vi "Get State.vi"(8 "error in (no error)":errorcluster, 11 "Spectrum Recorder in":refnum<class "Spectrum Recorder.lvclass">) -> (0 "error out":errorcluster, 3 "Spectrum Recorder out":refnum<class "Spectrum Recorder.lvclass">)   [LabVIEW 2016, in "Spectrum Recorder.lvclass"]
uses:
  Spectrum Recorder.lvclass
  Spectrum Recorder.lvclass/Spectrum Recorder.ctl
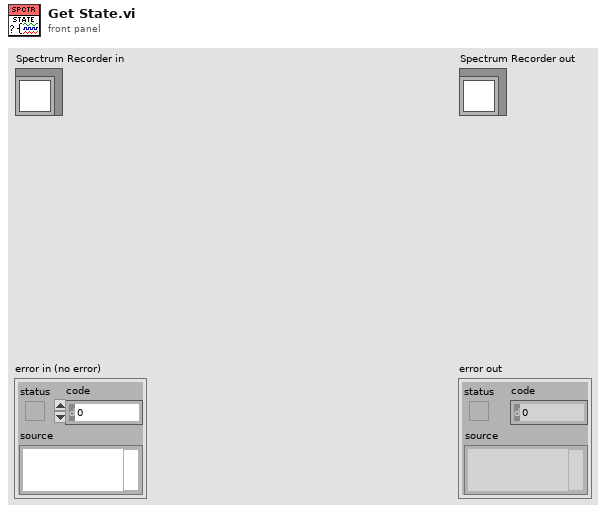
[diagram p1: front panel]
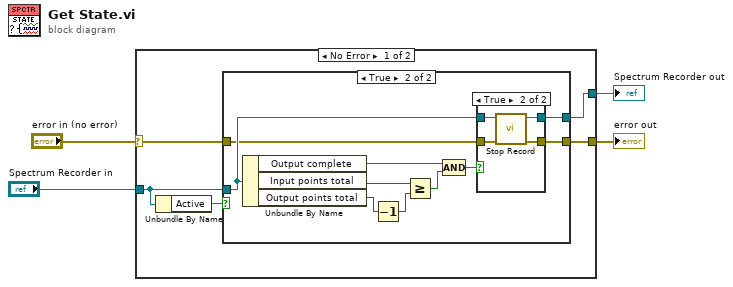
[diagram p0: block diagram]
diagram:
  n1 = case shown="No Error" "error in (no error)" {
    selector: "error in (no error)" -> [w6 w29]
    tunnel: [w5 w29] -> w3
    tunnel: [w7 w28] -> w1
    tunnel: "Spectrum Recorder in" -> [w8 w28]
    frame No Error {
      n2 = Unbundle By Name(w8) -> ("Active"=w9:bool)
      n3 = case shown="True" w9 {
        tunnel: w8 -> [w10 w17]
        tunnel: w6 -> [w11 w16]
        tunnel: [w11 w15] -> w5
        tunnel: [w10 w14] -> w7
        frame False {
        }
        frame True {
          n4 = Unbundle By Name(w17) -> ("Output complete"=w12:bool, "Input points total"=w20:i64, "Output points total"=w19:i64)
          n5 = Decrement(x=w19) -> (x-1=w13:i64)
          n6 = Greater Or Equal?(x=w20, y=w13) -> (x >= y?=w18:bool)
          n7 = Compound Arithmetic op=AND(w12, w18) -> (w21:bool)
          n8 = case shown="True" w21 {
            tunnel: w17 -> [w23 w27]
            tunnel: w16 -> [w22 w26]
            tunnel: [w22 w25] -> w15
            tunnel: [w23 w24] -> w14
            frame False {
            }
            frame True {
              n9 = call-dynamic "Stop Record.vi"("error in (no error)"=w26, "Spectrum Recorder in"=w27) -> ("error out"=w25:errorcluster, "Spectrum Recorder out"=w24:refnum<class "Spectrum Recorder.lvclass">)  [unwired: 8 in]
            }
          }
        }
      }
    }
    frame Error {
    }
  }
  "error out" <- w3
  "Spectrum Recorder out" <- w1
